vi "DriveGetSpeedDemand.vi"() -> (0 "ChassisSpeedDemand":T1 {"vOmega" format="%10.3f"; "vY" format="%10.3f"; "vX" format="%10.3f"}, 1 "vOmega":dbl, 2 "vY":dbl, 3 "vX":dbl)   [LabVIEW 2023]
doc: "Get speed demand variable for drive"
uses:
  <vilib>/Rock Robotics/WPI/ThirdParty/JAS_Junk/TrajLib/TypeDef/CHASSIS_SPEEDS.ctl
  DriveGlobal.vi
  <vilib>/Rock Robotics/WPI/ThirdParty/JAS_Junk/TrajLib/Trajectory_Library.lvlib
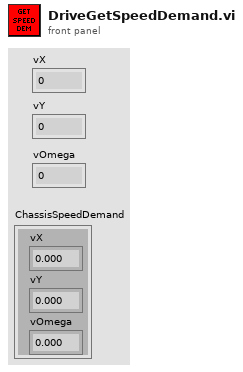
[diagram p1: front panel]
types:
  T1 = typedef "Trajectory_Library.lvlib/CHASSIS_SPEEDS.ctl" = cluster{"vX":dbl, "vY":dbl, "vOmega":dbl}
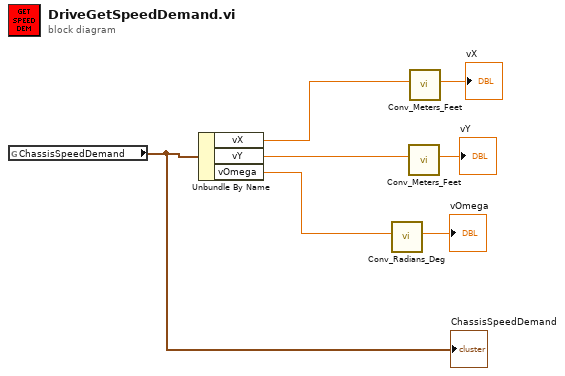
[diagram p0: block diagram]
diagram:
  n1 = global read "DriveGlobal.vi" "ChassisSpeedDemand"() -> (w7:T1)
  "ChassisSpeedDemand" <- w7
  n2 = Unbundle By Name(w7) -> ("vX"=w2:dbl, "vY"=w4:dbl, "vOmega"=w6:dbl)
  n3 = call <vilib>:"Conv_Radians_Deg.vi"("Radians"=w6) -> ("Degrees"=→"vOmega":dbl)  [unwired: 10 in]
  n4 = call <vilib>:"Conv_Meters_Feet.vi"("Meters"=w4) -> ("Feet"=→"vY":dbl)  [unwired: 10 in]
  n5 = call <vilib>:"Conv_Meters_Feet.vi"("Meters"=w2) -> ("Feet"=→"vX":dbl)  [unwired: 10 in]
